vi "Test Write.vi"() -> ()   [LabVIEW 2019, in "Control Experiment.lvclass"]
uses:
  Control Experiment.lvclass
  Control Experiment.lvclass/Control Experiment.ctl
  <vilib>/numeric/Random Number (Range) DBL.vi
  4aa6bf6a-cca5-4dbb-810b-5ed0c85cd02c.vi
  deaac86e-10e2-4daf-b676-4e754f80a0a7.vi
panel:
  out "error out":errorcluster
  in  "append?":bool=TRUE
  out "Data":string="SA03036H\nsweep Vsg:-150mV to 600mV, 1mV steps\nB: 7T to -7T\nVbg = -3.9V\nT: 50mK\n\nlockin\n\nI+/-: 2/3 3mV ac+ 250uV dc bias, 0.4 Hz\nV1+/-: 8/4\nV2+/- 6/28\nV3+/V3-: 27/8\nVsg: 1\nVbg :26\n\ntc 300ms order 2"
  out "Path":path
  in  "stop":bool
  in  "Experiment Folder":string="6H_IVcurves"
  in  "Experiment Comments":string="SA03036H\nsweep Vsg:-150mV to 600mV, 1mV steps\nB: 7T to -7T\nVbg = -3.9V\nT: 50mK\n\nlockin\n\nI+/-: 2/3 3mV ac+ 250uV dc bias, 0.4 Hz\nV1+/-: 8/4\nV2+/- 6/28\nV3+/V3-: 27/8\nVsg: 1\nVbg :26\n\ntc 300ms order 2"
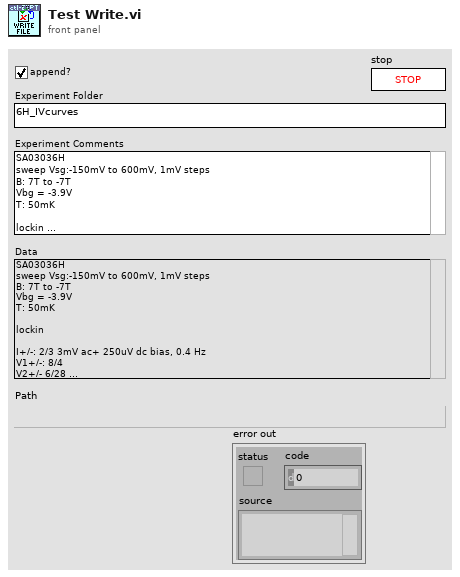
[diagram p1: front panel]
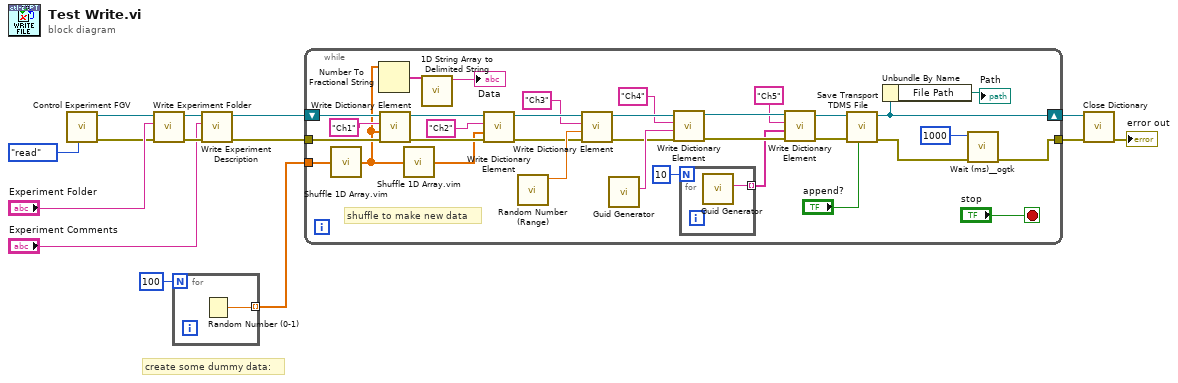
[diagram p0: block diagram]
diagram:
  # "create some dummy data:"
  n1 = call "Control Experiment FGV.vi"("Function"=enum16{"read", "write"}."read") -> ("error out"=w2:errorcluster, "Control Experiment.lvclass out"=w4:refnum<class "Control Experiment.lvclass">)  [unwired: 9 in]
  n2 = call "Write Experiment Folder.vi"("error in (no error)"=w2, "Experiment Folder"="Experiment Folder", "Control Experiment in"=w4) -> ("error out"=w13:errorcluster, "Control Experiment out"=w14:refnum<class "Control Experiment.lvclass">)  [unwired: 7 in]
  n3 = for {
    N: 100 -> [_]
    tunnel: [w15] -> w7 mode=indexing
    n4 = Random Number (0-1)() -> (number: 0 to 1=w15:dbl)
  }
  n5 = call "Write Experiment Description.vi"("error in (no error)"=w13, "Experiment Description"="Experiment Comments", "Control Experiment in"=w14) -> ("error out"=w11:errorcluster, "Control Experiment out"=w10:refnum<class "Control Experiment.lvclass">)  [unwired: 7 in]
  n6 = while {
    tunnel: w11 -> [w48]
    tunnel: w7 -> [w43]
    tunnel: [w38] -> w6
    shift-right: [w40] -> w5
    shift-left: w10 -> [w47]
    stop <- "stop" stop-if-true
    # "shuffle to make new data"
    n7 = call "Shuffle 1D Array.vim"("array"=w43) -> ("shuffled array"=w32:dbl[])  [unwired: 4 in]
    n8 = Number To Fractional String(number=w32) -> (F-format string=w42:string[])  [unwired: 3 in]
    n9 = call "Write Dictionary Element.vi"("error in (no error)"=w48, "value"=w32, "key"="Ch1", "Control Experiment in"=w47) -> ("error out"=w34:errorcluster, "Control Experiment out"=w35:refnum<class "Control Experiment.lvclass">)  [unwired: 6 in]
    n10 = call "Shuffle 1D Array.vim"("array"=w32) -> ("shuffled array"=w31:dbl[])  [unwired: 4 in]
    n11 = call <vilib>:"1D String Array to Delimited String.vi"("string array"=w42) -> ("delimited string"=→"Data":string)  [unwired: 10 in]
    n12 = call "Write Dictionary Element.vi"("error in (no error)"=w34, "value"=w31, "key"="Ch2", "Control Experiment in"=w35) -> ("error out"=w27:errorcluster, "Control Experiment out"=w30:refnum<class "Control Experiment.lvclass">)  [unwired: 6 in]
    n13 = call-poly <vilib>:"Random Number (Range).vi"() -> ("number"=w28:dbl)  [unwired: 11 in]
    n14 = call "Write Dictionary Element.vi"("error in (no error)"=w27, "value"=w28, "key"="Ch3", "Control Experiment in"=w30) -> ("error out"=w22:errorcluster, "Control Experiment out"=w26:refnum<class "Control Experiment.lvclass">)  [unwired: 6 in]
    n15 = call <vilib>:"Guid Generator.vi"() -> ("GUID"=w24:string)  [unwired: 10 in, 1 out]
    n16 = call "Write Dictionary Element.vi"("error in (no error)"=w22, "value"=w24, "key"="Ch4", "Control Experiment in"=w26) -> ("error out"=w19:errorcluster, "Control Experiment out"=w23:refnum<class "Control Experiment.lvclass">)  [unwired: 6 in]
    n17 = for {
      N: 10 -> [_]
      tunnel: [w49] -> w16 mode=indexing
      n18 = call <vilib>:"Guid Generator.vi"() -> ("GUID"=w49:string)  [unwired: 10 in, 1 out]
    }
    n19 = call "Write Dictionary Element.vi"("error in (no error)"=w19, "value"=w16, "key"="Ch5", "Control Experiment in"=w23) -> ("error out"=w18:errorcluster, "Control Experiment out"=w17:refnum<class "Control Experiment.lvclass">)  [unwired: 6 in]
    n20 = call "Save Transport TDMS File.vi"("append?"="append?", "error in (no error)"=w18, "Control Experiment in"=w17) -> ("error out"=w39:errorcluster, "Control Experiment out"=w40:refnum<class "Control Experiment.lvclass">)  [unwired: 7 in]
    n21 = Unbundle By Name(w40) -> ("File Path"=→"Path":path)
    n22 = call <userlib>:"Wait (ms)__ogtk.vi"("error in (no error)"=w39, "milliseconds to wait"=u32 1000) -> ("error out"=w38:errorcluster)  [unwired: 8 in, 1 out]
  }
  n23 = call "Close Dictionary.vi"("error in (no error)"=w6, "Control Experiment in"=w5) -> ("error out"=→"error out":errorcluster)  [unwired: 8 in, 1 out]
